vi "json_parse_object.vi"(8 "error in (no error)":errorcluster, 10 "parent key":string, 11 "data":string) -> (0 "error out":errorcluster, 2 "pairs":cluster{"key":string, "value":variant}[](array[cluster]), 3 "remaining data":string)   [LabVIEW 2017]
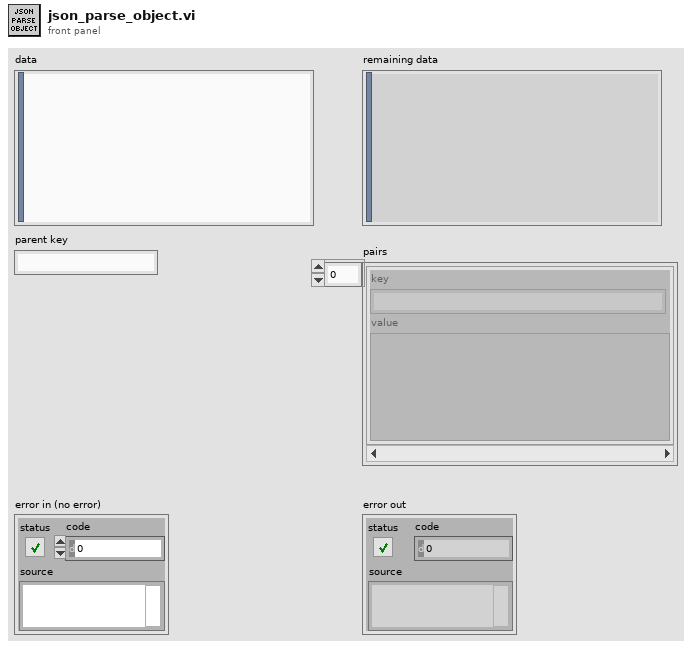
[diagram p1: front panel]
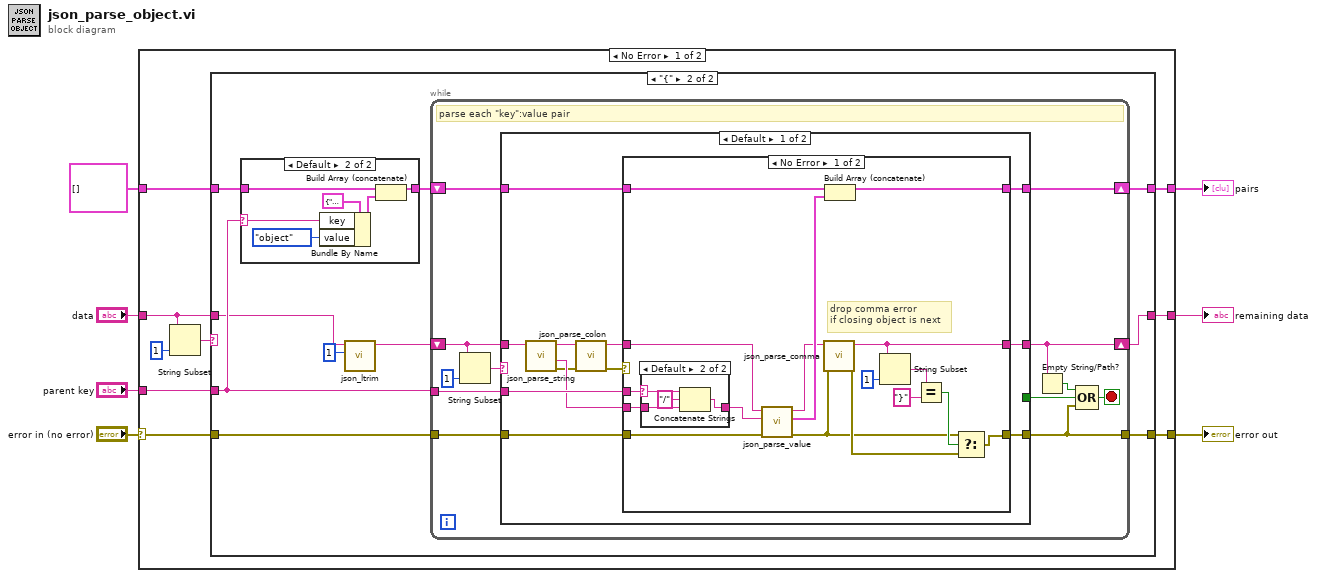
[diagram p0: block diagram]
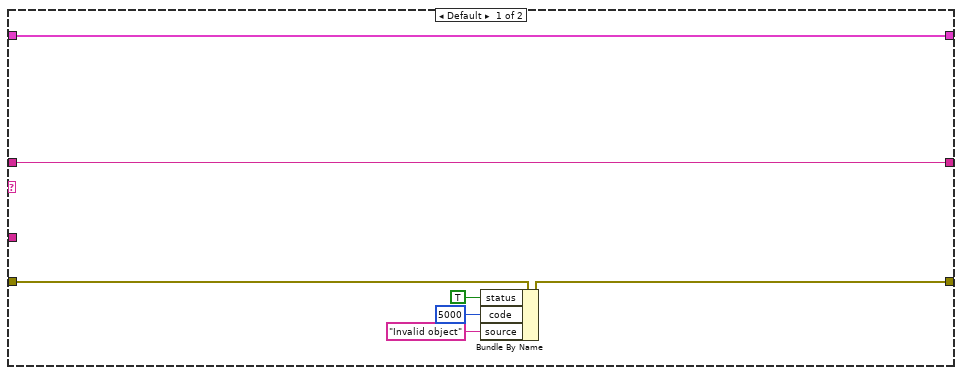
[diagram p2: hidden frame]
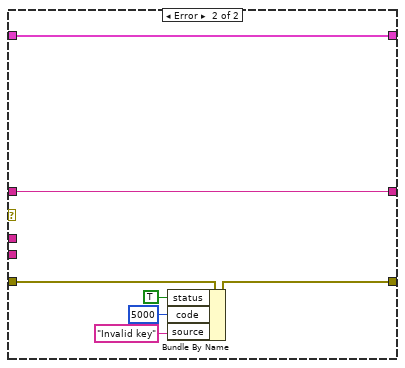
[diagram p5: hidden frame]
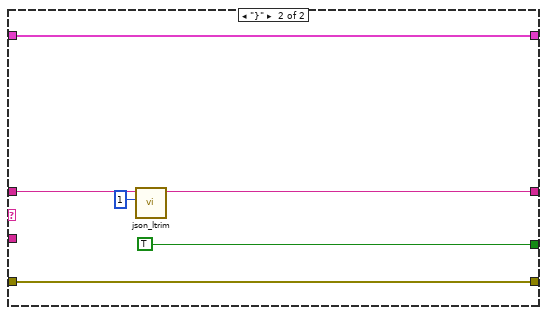
[diagram p6: hidden frame]
diagram:
  n1 = case shown="No Error" "error in (no error)" {
    selector: "error in (no error)" -> [w15 w102]
    tunnel: [w16 w101] -> w7
    tunnel: [w14 w102] -> w5
    tunnel: "parent key" -> [w13 _]
    tunnel: [w12 w100] -> w3
    tunnel: cluster{"key":string, "value":variant}[] [] ("appended array") -> [w11 w101]
    tunnel: "data" -> [w10 w100]
    frame No Error {
      n2 = String Subset(string=w10, length (rest)=1 ("length (rest)")) -> (substring=w9:string)  [unwired: 1 in]
      n3 = case shown="\"{\"" w9 {
        tunnel: w10 -> [w23 w24]
        tunnel: [w23 w31] -> w12
        tunnel: [w22 w30] -> w16
        tunnel: w11 -> [w22 w29]
        tunnel: w15 -> [w21 w33]
        tunnel: [w20 w32] -> w14
        tunnel: w13 -> [_ w28]
        frame Default {
          n4 = Bundle By Name(cluster=w21, "status"=TRUE, "code"=5000, "source"="Invalid object") -> (w20:errorcluster)
        }
        frame "{" {
          n5 = case shown="Default" w28 {
            selector: w28 -> [_ w37]
            tunnel: [w34 w38] -> w27
            tunnel: w29 -> [w34 w36]
            frame "" {
            }
            frame Default {
              n6 = Bundle By Name(cluster=cluster{"key":string, "value":variant} {"key"="", "value"=variant} ("pair"), "key"=w37, "value"=enum8{"object"}."object" ("object")) -> (w39:cluster{"key":string, "value":variant})
              n7 = Build Array (concatenate)(w36, w39) -> (w38:cluster{"key":string, "value":variant}[])
            }
          }
          n8 = call "json_ltrim.vi"("offset (0)"=1, "data"=w24) -> ("left trim whitespace"=w25:string)  [unwired: 9 in]
          n9 = while {
            shift-right: [w52] -> w30
            shift-left: w27 -> [w51]
            shift-right: [w45] -> w31
            shift-left: w25 -> [w43]
            tunnel: w33 -> [w50]
            tunnel: [w46] -> w32
            tunnel: w28 -> [w49]
            stop <- w47 stop-if-true
            # "parse each \"key\":value pair"
            n10 = String Subset(string=w43, length (rest)=1 ("length (rest)")) -> (substring=w42:string)  [unwired: 1 in]
            n11 = case shown="Default" w42 {
              tunnel: [_ TRUE] -> w48
              tunnel: [w60 w98] -> w52
              tunnel: w51 -> [w59 w98]
              tunnel: w43 -> [w64 w95]
              tunnel: [w63 w94] -> w45
              tunnel: w50 -> [w53 w97]
              tunnel: [w61 w97] -> w46
              tunnel: w49 -> [w58 _]
              frame Default {
                n12 = call "json_parse_string.vi"("data"=w64) -> ("error out"=w55:errorcluster, "raw_string"=w57:string, "remaining data"=w62:string)  [unwired: 7 in, 1 out]
                n13 = call "json_parse_colon.vi"("error in (no error)"=w55, "data"=w62) -> ("error out"=w54:errorcluster, "remaining data"=w56:string)  [unwired: 8 in]
                n14 = case shown="No Error" w54 {
                  tunnel: [w72 w87] -> w63
                  tunnel: [w66 w92] -> w61
                  tunnel: [w77 w88] -> w60
                  tunnel: w59 -> [w78 w88]
                  tunnel: w58 -> [w81 _]
                  tunnel: w57 -> [w80 _]
                  tunnel: w56 -> [w75 w87]
                  tunnel: w53 -> [w79 w93]
                  frame No Error {
                    # "drop comma error\nif closing object is next"
                    n15 = case shown="Default" w81 {
                      selector: w81 -> [_ w86]
                      tunnel: w80 -> [w82 w85]
                      tunnel: [w82 w84] -> w74
                      frame "" {
                      }
                      frame Default {
                        n16 = Concatenate Strings(w86, "/" ("format string"), w85) -> (w84:string)
                      }
                    }
                    n17 = call "json_parse_value.vi"("error in (no error)"=w79, "key"=w74, "data"=w75) -> ("error out"=w65:errorcluster, "pairs"=w76:cluster{"key":string, "value":variant}[], "remaining data"=w73:string)  [unwired: 6 in]
                    n18 = call "json_parse_comma.vi"("error in (no error)"=w65, "data"=w73) -> ("error out"=w67:errorcluster, "remaining data"=w72:string)  [unwired: 8 in]
                    n19 = Build Array (concatenate)(w78, w76) -> (w77:cluster{"key":string, "value":variant}[])
                    n20 = String Subset(string=w72, length (rest)=1 ("length (rest)")) -> (substring=w70:string)  [unwired: 1 in]
                    n21 = Equal?(x=w70, y="}") -> (x = y?=w68:bool)
                    n22 = Select(t=w65, s=w68, f=w67) -> (s? t:f=w66:errorcluster)
                  }
                  frame Error {
                    n23 = Bundle By Name(cluster=w93, "status"=TRUE, "code"=5000, "source"="Invalid key") -> (w92:errorcluster)
                  }
                }
              }
              frame "}" {
                n24 = call "json_ltrim.vi"("offset (0)"=1, "data"=w95) -> ("left trim whitespace"=w94:string)  [unwired: 9 in]
              }
            }
            n25 = Empty String/Path?(string/path=w45) -> (empty?=w44:bool)
            n26 = Compound Arithmetic op=OR(w44, w48, w46) -> (w47:bool)
          }
        }
      }
    }
    frame Error {
    }
  }
  "remaining data" <- w3
  "pairs" <- w7
  "error out" <- w5
